vi "PXI Attens to Multipliers (1D).vi"(8 "error in (no error)":errorcluster, 11 "Array of Attens":dbl[](array[numeric])) -> (0 "error out":errorcluster, 3 "Multiplier setting":dbl[](array[numeric])=[1.0, 0.001, 1.0, 1.0, 1.0, 1.0, 1.0, 1.0])   [LabVIEW 2020]
doc: "Set multiplier values by writing the config file.\nIt also changes the multiplier global variable."
uses:
  Utility VIs/Math VIs/dB to Linear (scalar).vi
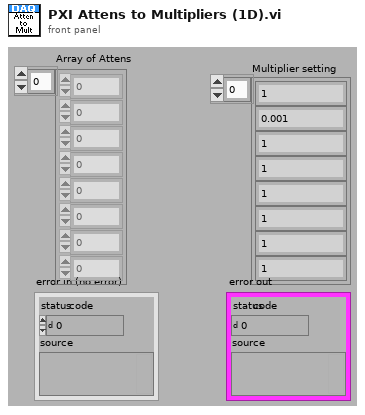
[diagram p1: front panel]
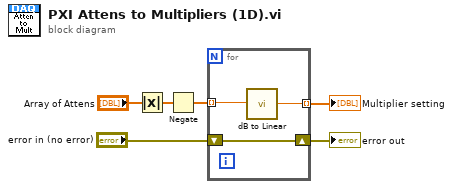
[diagram p0: block diagram]
diagram:
  n1 = Absolute Value(x="Array of Attens") -> (abs(x)=w2:dbl[])
  n2 = Negate(x=w2) -> (-x=w1:dbl[])
  n3 = for {
    tunnel: [w7] -> w4 mode=indexing
    shift-right: [w9] -> w6
    shift-left: "error in (no error)" -> [w9]
    tunnel: w1 -> [w8] mode=indexing
    n4 = call-poly "dB to Linear.vi"("dB"=w8) -> ("linear"=w7:dbl)
  }
  "Multiplier setting" <- w4
  "error out" <- w6
